vi "Write_Preproc_Session_Ref.vi"(8 "error in (no error)":errorcluster, 10 "Session_ref":refnum<k35>, 11 "Python in":refnum<class "Python.lvclass">) -> (0 "error out":errorcluster, 3 "Python out":refnum<class "Python.lvclass">)   [LabVIEW 2020, in "Python.lvclass"]
uses:
  Python.lvclass
  Python.lvclass/Python.ctl
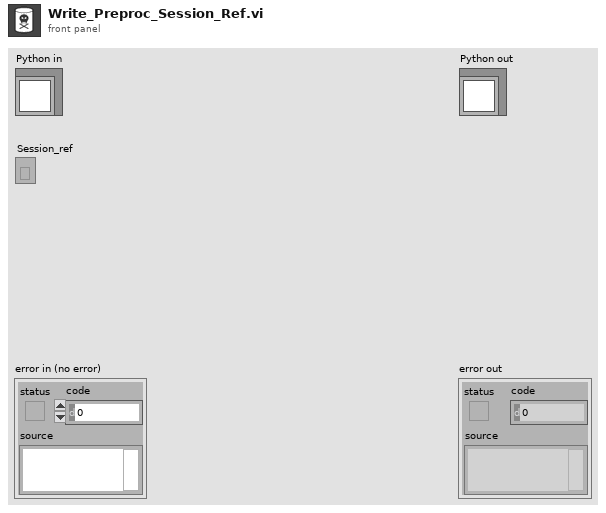
[diagram p1: front panel]
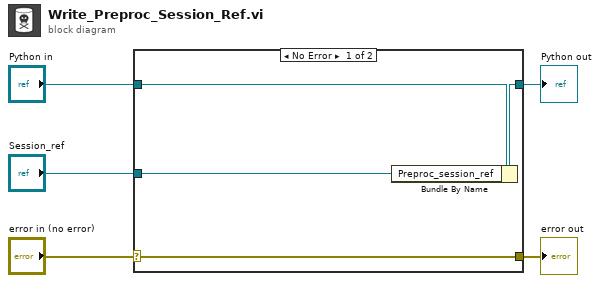
[diagram p0: block diagram]
diagram:
  n1 = case shown="No Error" "error in (no error)" {
    selector: "error in (no error)" -> [w9 w10]
    tunnel: [w9 w10] -> w4
    tunnel: [w7 w11] -> w2
    tunnel: "Python in" -> [w8 w11]
    tunnel: "Session_ref" -> [w6 _]
    frame No Error {
      n2 = Bundle By Name(cluster=w8, "Preproc_session_ref"=w6) -> (w7:refnum<class "Python.lvclass">)
    }
    frame Error {
    }
  }
  "error out" <- w4
  "Python out" <- w2
